vi "3.6-Act Arbitrator.vi"   [LabVIEW 2010]
uses:
  <vilib>/Platform/TimedLoop/XDataNode/wakeup.ctl
  <vilib>/Platform/TimedLoop/XDataNode/XDNodeRunTimeDep.lvlib
  <vilib>/Platform/TimedLoop/XDataNode/nitl_modes.ctl
  <vilib>/Platform/TimedLoop/XDataNode/timing_clust.ctl
  <vilib>/Platform/TimedLoop/XDataNode/XDataNode.xnode
  3.0-Global.vi
  <vilib>/rvi/interface/nirviReadWriteControl/nirviReadWriteControl.xnode
  1-Hindbrain.vi
  4-High Neurons/4.1-FPGA VI Typedef.ctl
  2-Low Neurons/2.1-Act Command Typedef.ctl
  <vilib>/RVI Host/nirviSupport.llb/nirviErrorClusterFromErrorCode.vi
  <vilib>/rvi/errors/niLvFpgaWhatHappensToTopLevelVI.ctl
  <vilib>/rvi/interface/common/niFpgaNodeNameForErrorReporting.ctl
  <vilib>/rvi/errors/niLvFpgaAdjustHostInterfaceError.vi
types:
  T1 = typedef "XDNodeRunTimeDep.lvlib/timing_clust.ctl" = cluster{"Expected End [f-1]":u64, "Actual End [f-1]":u64, "Finished Late? [f-1]":bool, "Expected End [i-1]":u64, "Actual End [i-1]":u64, "Finished Late? [i-1]":bool, "Expected Start [i]":u64, "Actual Start [i]":u64, "Expected Start [f]":u64, "Actual Start [f]":u64, "Source Name":string, "Structure Name":string, "Period":i64, "Deadline":i64, "Offset":i64, "Start":i64, "Priority":i32, "Timeout":i32, "Mode":T2, "Wakeup Reason":T3, "Error":errorcluster, "Source Type":string, "Secondary Source Type":string, "Global End Time":u64, "Global Start Time":u64, "Frame Duration":u64, "Iteration Duration":u64, "Assigned CPU":i32, "I/O Scan Engine Mode":u32}
  T2 = typedef "XDNodeRunTimeDep.lvlib/nitl_modes.ctl" = enum32{"No Change", "Process missed periods, maintain original phase", "Discard missed periods, maintain original phase", "Process missed periods, ignore original phase", "Discard missed periods, ignore original phase"}
  T3 = typedef "XDNodeRunTimeDep.lvlib/wakeup.ctl" = enum32{"Normal", "Aborted", "Asynchronous wakeup", "Timing source error", "Timed loop error", "Timeout"}
  T4 = typedef "2.1-Act Command Typedef.ctl" = cluster{"Steering Integer Setpoint":i16, "Drive Speed Integer Setpoint":i16, "Lidar Position Integer Setpoint":i16, "Inhibit All Motors":bool}
  T5 = typedef "niFpgaNodeNameForErrorReporting.ctl" = enum16{"Open FPGA VI Reference", "Read/Write Control", "Invoke Method: Abort", "Invoke Method: Acknowledge IRQ", "Invoke Method: Download", "Invoke Method: FIFO.Configure", "Invoke Method: FIFO.Read", "Invoke Method: FIFO.Start", "Invoke Method: FIFO.Stop", "Invoke Method: FIFO.Write", "Invoke Method: Reset", "Invoke Method: Run", "Invoke Method: Wait on IRQ", "Close FPGA VI Reference"}
  T6 = typedef "niLvFpgaWhatHappensToTopLevelVI.ctl" = enum16{"top level VI scripted behind XNode", "top level VI inlined behind XNode"}
  T7 = typedef "4.1-FPGA VI Typedef.ctl" = refnum<k20>
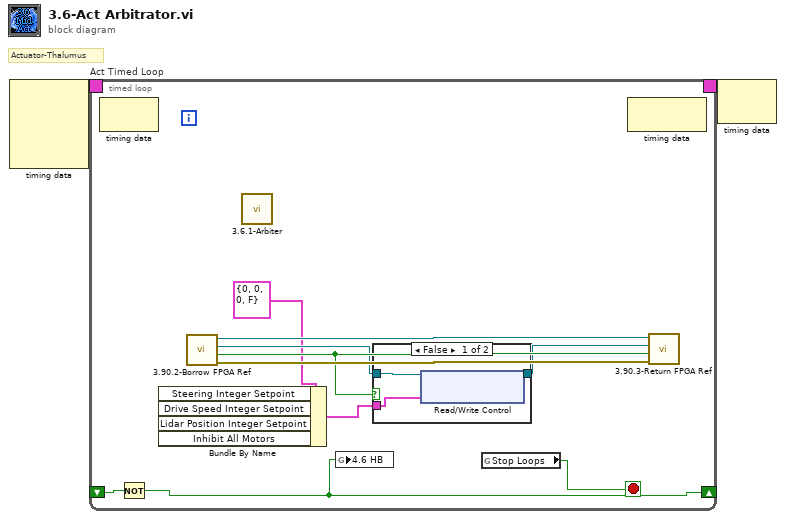
[diagram p0: block diagram]
diagram:
  # "Actuator-Thalumus"
  n1 = node-c288 ("Input Node")() -> (w2:T1)  [unwired: 4 in]
  n2 = timed-loop "Act Timed Loop" {
    timing: w2 -> [_]
    timing-out: [_] -> w1
    shift-right: [w8] -> _
    shift-left: _ -> [w12]
    stop <- w9 stop-if-true
    n3 = node-c288() -> ()  [unwired: 1 in, 1 out]
    n4 = Not(x=w12) -> (.not. x?=w8:bool)
    n5 = Bundle By Name(cluster=T4 {"Steering Integer Setpoint"=0, "Drive Speed Integer Setpoint"=0, "Lidar Position Integer Setpoint"=0, "Inhibit All Motors"=FALSE} ("2.1 Act Command")) -> (w3:T4)  [unwired: 4 in]
    n6 = call "3.90.2-Borrow FPGA Ref.vi"() -> ("error out"=w10:errorcluster, "Failed to Obtain Ref"=w7:bool, "element"=w6:T7, "FPGA Ref"=w11:refnum<queue>)  [unwired: 4 in]
    n7 = call "3.6.1-Arbiter.vi"() -> ()  [unwired: 12 in, 4 out]
    n8 = global write "3.0-Global.vi" "4.6 HB"(w8) -> ()
    n9 = case shown="False" w7 {
      tunnel: w6 -> [w15 w37]
      tunnel: [w14 w37] -> w5
      tunnel: w3 -> [w13 _]
      frame False {
        n10 = xnode "Read/Write Control"("FPGA VI Reference In"=w15, "2.1 Act Command"=w13) -> ("FPGA VI Reference Out"=w14:T7)  [unwired: 1 in, 1 out]
      }
      frame True {
      }
    }
    n11 = global read "3.0-Global.vi" "Stop Loops"() -> (w9:bool)
    n12 = node-c288() -> ()  [unwired: 1 in, 1 out]
    n13 = call "3.90.3-Return FPGA Ref.vi"("error in"=w10, "Failed to Obtain Ref"=w7, "element"=w5, "FPGA Ref"=w11) -> ()  [unwired: 1 out]
  }
  n14 = node-c288(w1) -> ()  [unwired: 1 out]
